vi "Is Camera Supported (SubVI).vi"(8 "error in (no error)":errorcluster, 11 "Refnum in":T1) -> (0 "error out":errorcluster, 2 "Pixel Format":string[](array[string]), 3 "Refnum out":T1)   [LabVIEW 2023]
uses:
  <vilib>/userDefined/High Color/IMAQdx.ctl
  <resource>/objmgr/imaqdx.rc
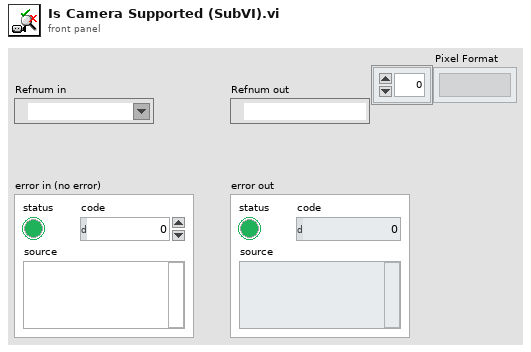
[diagram p1: front panel]
types:
  T1 = typedef "IMAQdx.ctl" = refnum<k21>
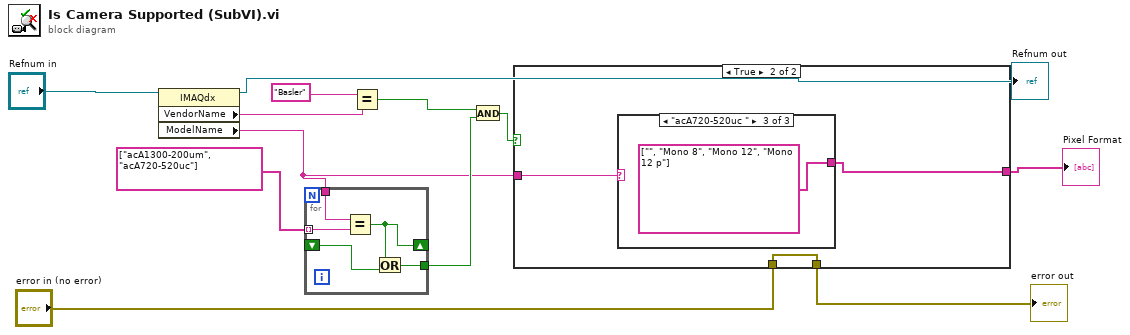
[diagram p0: block diagram]
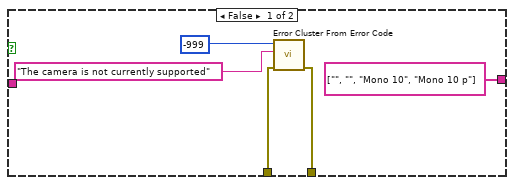
[diagram p2: hidden frame]
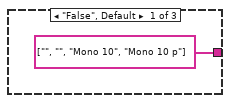
[diagram p3: hidden frame]
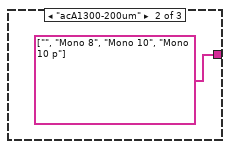
[diagram p4: hidden frame]
diagram:
  n1 = property class="IMAQdx"(reference="Refnum in") -> (reference out=→"Refnum out":T1, "VendorName"=w10:string, "ModelName"=w2:string)  [unwired: 1 in, 1 out]
  n2 = for {
    tunnel: string[] ["acA1300-200um", "acA720-520uc"] -> [w17] mode=indexing
    tunnel: w2 -> [w16]
    shift-right: [w14] -> _
    shift-left: _ -> [w15]
    tunnel: [w13] -> w5
    n3 = Equal?(x=w16, y=w17) -> (x = y?=w14:bool)
    n4 = Or(x=w14, y=w15) -> (x .or. y?=w13:bool)
  }
  n5 = Equal?(x="Basler", y=w10) -> (x = y?=w7:bool)
  n6 = And(x=w7, y=w5) -> (x .and. y?=w8:bool)
  n7 = case shown="True" w8 {
    tunnel: "error in (no error)" -> [w20 w25]
    tunnel: [w19 w25] -> w3
    tunnel: w2 -> [_ w24]
    tunnel: [string[] ["", "", "Mono 10", "Mono 10 p"] w23] -> w1
    frame False {
      n8 = call <vilib>:"Error Cluster From Error Code.vi"("error in (no error)"=w20, "error message (\"\")"="The camera is not currently supported" ("source"), "error code (0)"=-999 ("code")) -> ("error out"=w19:errorcluster)  [unwired: 6 in]
    }
    frame True {
      n9 = case shown="\"acA720-520uc \"" w24 {
        tunnel: [string[] ["", "", "Mono 10", "Mono 10 p"] string[] ["", "Mono 8", "Mono 10", "Mono 10 p"] string[] ["", "Mono 8", "Mono 12", "Mono 12 p"]] -> w23
        frame "False", Default {
        }
        frame "acA1300-200um" {
        }
        frame "acA720-520uc " {
        }
      }
    }
  }
  "error out" <- w3
  "Pixel Format" <- w1
